vi "Teardown.vi"(6 "Delete Temporary File":bool=TRUE, 8 "Error In":errorcluster, 10 "Temporary File":string, 11 "SFTP":refnum<class "SFTP.lvclass">) -> (0 "Error Out":errorcluster)   [LabVIEW 2018, in "Tests.lvlib" / "SFTP File.lvlib"]
uses:
  SFTP File.lvlib
  src/Toolkit/SFTP/SFTP.lvclass
  src/Toolkit/Session/Support/Destroy to SSH.vi
  src/Toolkit/Session/Session.lvclass
  src/Toolkit/SSH/SSH.lvclass
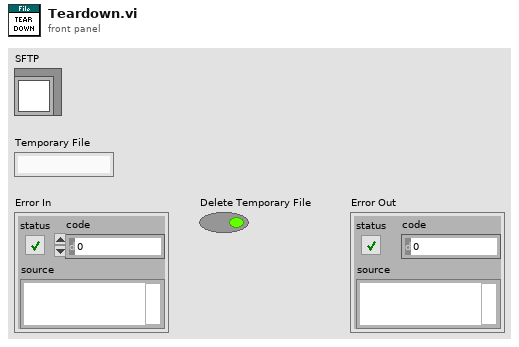
[diagram p1: front panel]
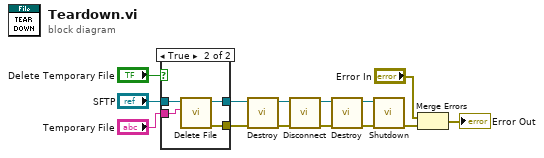
[diagram p0: block diagram]
diagram:
  n1 = case shown="True" "Delete Temporary File" {
    tunnel: "SFTP" -> [w15 w19]
    tunnel: [w15 w18] -> w4
    tunnel: [_ w17] -> w3
    tunnel: "Temporary File" -> [_ w16]
    frame False {
    }
    frame True {
      n2 = call "Delete File.vi"("Remote Path"=w16, "SFTP In"=w19) -> ("Error Out"=w17:errorcluster, "SFTP Out"=w18:refnum<class "SFTP.lvclass">)  [unwired: 8 in]
    }
  }
  n3 = call "Destroy.vi"("Error In"=w3, "SFTP"=w4) -> ("Error Out"=w14:errorcluster, "Session"=w6:refnum<class "Session.lvclass">)  [unwired: 8 in]
  n4 = call "Disconnect.vi"("Error In"=w14, "Session In"=w6) -> ("Error Out"=w13:errorcluster, "Sesssion Out"=w12:refnum<class "Session.lvclass">)  [unwired: 8 in]
  n5 = call-poly "Destroy.vi"("Error In"=w13, "Session"=w12) -> ("Error Out"=w10:errorcluster, "SSH"=w9:refnum<class "SSH.lvclass">)  [unwired: 8 in]
  n6 = call "Shutdown.vi"("Error In"=w10, "SSH"=w9) -> ("Error Out"=w11:errorcluster)  [unwired: 9 in]
  n7 = Merge Errors("Error In", w11) -> (→"Error Out":errorcluster)
